vi "h.SYSTEM.GetVersion.vi"(8 "error in":errorcluster, 11 "Connection ID In":refnum<k5>) -> (0 "error out":errorcluster, 1 "FPGA Version":string, 2 "Firmware Version":string, 3 "Connection ID Out":refnum<k5>, 4 "h.Library Version":string)   [LabVIEW 2016, in "h.Library.lvlib"]
doc: "Use this VI to retrieve the version number of the different Hyperion firmware modules.\n\n<b>Connection ID</b> - is a network connection refnum that uniquely identifies the TCP connection\n<b>Timeout</b> - specifies the maximum amount of time, in milliseconds, for the function to complete\n<b>error in</b> - describes error conditions that occur before this node runs. This input provides standard error functionality\n<b>Connection ID out</b> - returns the same value as connection ID\n<b>Firmware Version</b> - version number of the instrument's embedded firmware\n<b>FPGA Version</b> - version number of the instrument's FPGA firmware\n<b>h.Library Version</b> - LabView Hyperion API library (h.Library.lvlib) version\n<b>error out</b> - contains error information. This output provides standard error out functionality."
uses:
  h.Library.lvlib
panel:
  # "Hyperion Firmware Versions"
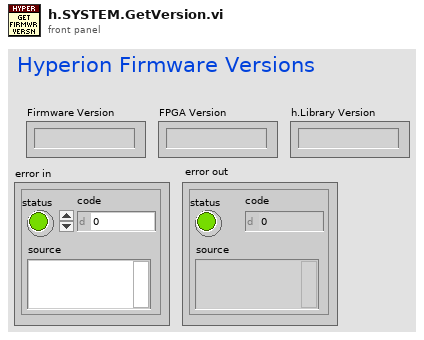
[diagram p1: front panel]
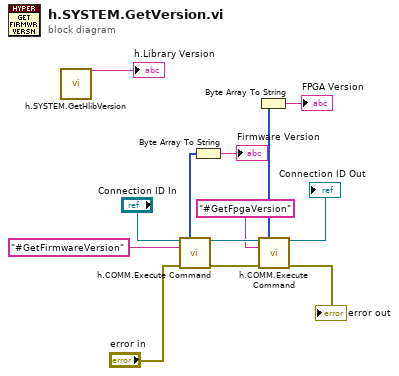
[diagram p0: block diagram]
diagram:
  n1 = call "h.SYSTEM.GetHlibVersion.vi"() -> ("h.Library Version"=→"h.Library Version":string)  [unwired: 1 in]
  n2 = call "h.COMM.Execute Command.vi"("Connection ID"="Connection ID In", "Command"="#GetFirmwareVersion", "error in"="error in") -> ("Content"=w4:u8[], "Connection ID out"=w9:refnum<k5>, "error out"=w8:errorcluster)  [unwired: 5 in, 5 out]
  n3 = Byte Array To String(unsigned byte array=w4) -> (string=→"Firmware Version":string)
  n4 = call "h.COMM.Execute Command.vi"("Connection ID"=w9, "Command"="#GetFpgaVersion", "error in"=w8) -> ("Content"=w1:u8[], "Connection ID out"=→"Connection ID Out":refnum<k5>, "error out"=→"error out":errorcluster)  [unwired: 5 in, 5 out]
  n5 = Byte Array To String(unsigned byte array=w1) -> (string=→"FPGA Version":string)
